vi "Abort Status Check.vi"(8 "error in (no error)":errorcluster, 11 "Guardian in":refnum<class "Guardian.lvclass">) -> (0 "error out":errorcluster, 3 "Guardian out":refnum<class "Guardian.lvclass">)   [LabVIEW 2026, in "TALOS.lvlib" / "Guardian.lvlib" / "Guardian.lvclass"]
doc: "This VI is called periodically to check the health status of ABORT and its unicity."
uses:
  Guardian.lvclass
  C:/LabVIEW Code/TALOS/talos/Ancestor/Ancestor/Ancestor.lvclass
  C:/LabVIEW Code/TALOS/builds/Actor Framework PPL/Actor Framework.lvlibp/1abvi3w/vi.lib/ActorFramework/Actor/Actor.lvclass
  Guardian.lvclass/Guardian.ctl
  Ancestor/Ancestor/Ancestor.lvclass/Ancestor.ctl
  Classes/Speedometer/Speedometer.lvclass/Speedometer.ctl
  Guardian Messages/Message to Other Guardian Msg/Message to Other Guardian Msg.lvclass/Message to Other Guardian Msg.ctl
  Guardian Messages/TCP-SV Message Interpreter Msg/TCP-SV Message Interpreter Msg.lvclass/TCP-SV Message Interpreter Msg.ctl
  4755b682-1248-473b-8cd2-dfaaffe09b65.vi
  cbc8a120-93e6-4d44-b253-7cefa591677c.vi
  3ae19a6a-4145-421c-a6fa-2879faec311c.vi
  Support VIs/Generate Error.vi
  <vilib>/Utility/High Resolution Relative Seconds.vi
  Broadcast to Guardians.vi
  FGV/Error Memory/Get Error Description.vi
  Support VIs/Get PC name.vi
  Support VIs/Get Class Name.vi
  Guardian Messages/Message to Other Guardian Msg/Send Message to Other Guardian.vi
  Support VIs/Search Array of Strings.vi
  Guardian Messages/TCP-SV Message Interpreter Msg/Send TCP-SV Message Interpreter.vi
  FGV/Error Memory/Error Memory Core.vi
  <vilib>/AdvancedString/Delimited String to 1D String Array.vi
  <vilib>/AdvancedString/Delimited String to 1D String Array (string).vi
  Support VIs/Circus Root Path.vi
  FGV/Error Memory/Error Crt Lvl checker.vi
  FGV/Error Memory/Error Memory Core.vi/40c8088d-b597-4017-91af-faa98e00292e.vi
  FGV/Error Memory/Error Memory Core.vi/d4a3ab98-063c-4e44-b43d-fbdcfe6c2be2.vi
  Support VIs/Global Memory.vi
  <vilib>/Utility/LVClass/Get LV Class Name.vi
  Support VIs/Is in Packed Library.vi
  Support VIs/TALOS Root path.vi
  Support VIs/Read CSV worksheet.vi
  Support VIs/Global Constants.vi
  <vilib>/Utility/error.llb/General Error Handler.vi
  <vilib>/Utility/config.llb/Open Config Data.vi
  <vilib>/Utility/config.llb/Get Section Names.vi
  <vilib>/Utility/config.llb/Get Key Names.vi
  <vilib>/Utility/config.llb/Read Key.vi
  <vilib>/Utility/config.llb/Read Key (String).vi
  <vilib>/Utility/config.llb/Close Config Data.vi
  Pat message.vi
  Support VIs/Circus Critical PCs List.vi
  builds/Actor Framework PPL/Actor Framework.lvlibp/1abvi3w/vi.lib/ActorFramework/Actor/Read Self Enqueuer.vi
  builds/Actor Framework PPL/Actor Framework.lvlibp/1abvi3w/vi.lib/ActorFramework/Message Enqueuer/Enqueue.vi
  Support VIs/Error Log.vi
  Support VIs/System Log.vi
  Ancestor/Ancestor/Ancestor.lvclass
  <vilib>/Comparison/Equal/Equal Functor/Equal Functor.lvclass
  Classes/Speedometer/Speedometer.lvclass
  <vilib>/Comparison/Less/Less Functor/Less Functor.lvclass
  Guardian Messages/Message to Other Guardian Msg/Message to Other Guardian Msg.lvclass
  Guardian Messages/TCP-SV Message Interpreter Msg/TCP-SV Message Interpreter Msg.lvclass
  Classes/Guardian List/Guardian List.lvclass
  TALOS.lvlib
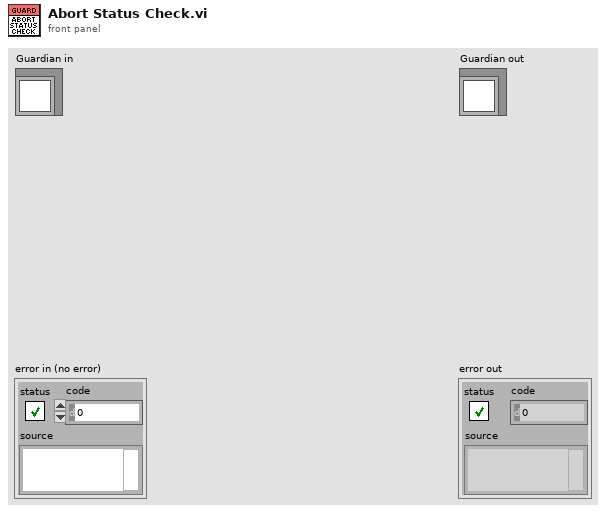
[diagram p1: front panel]
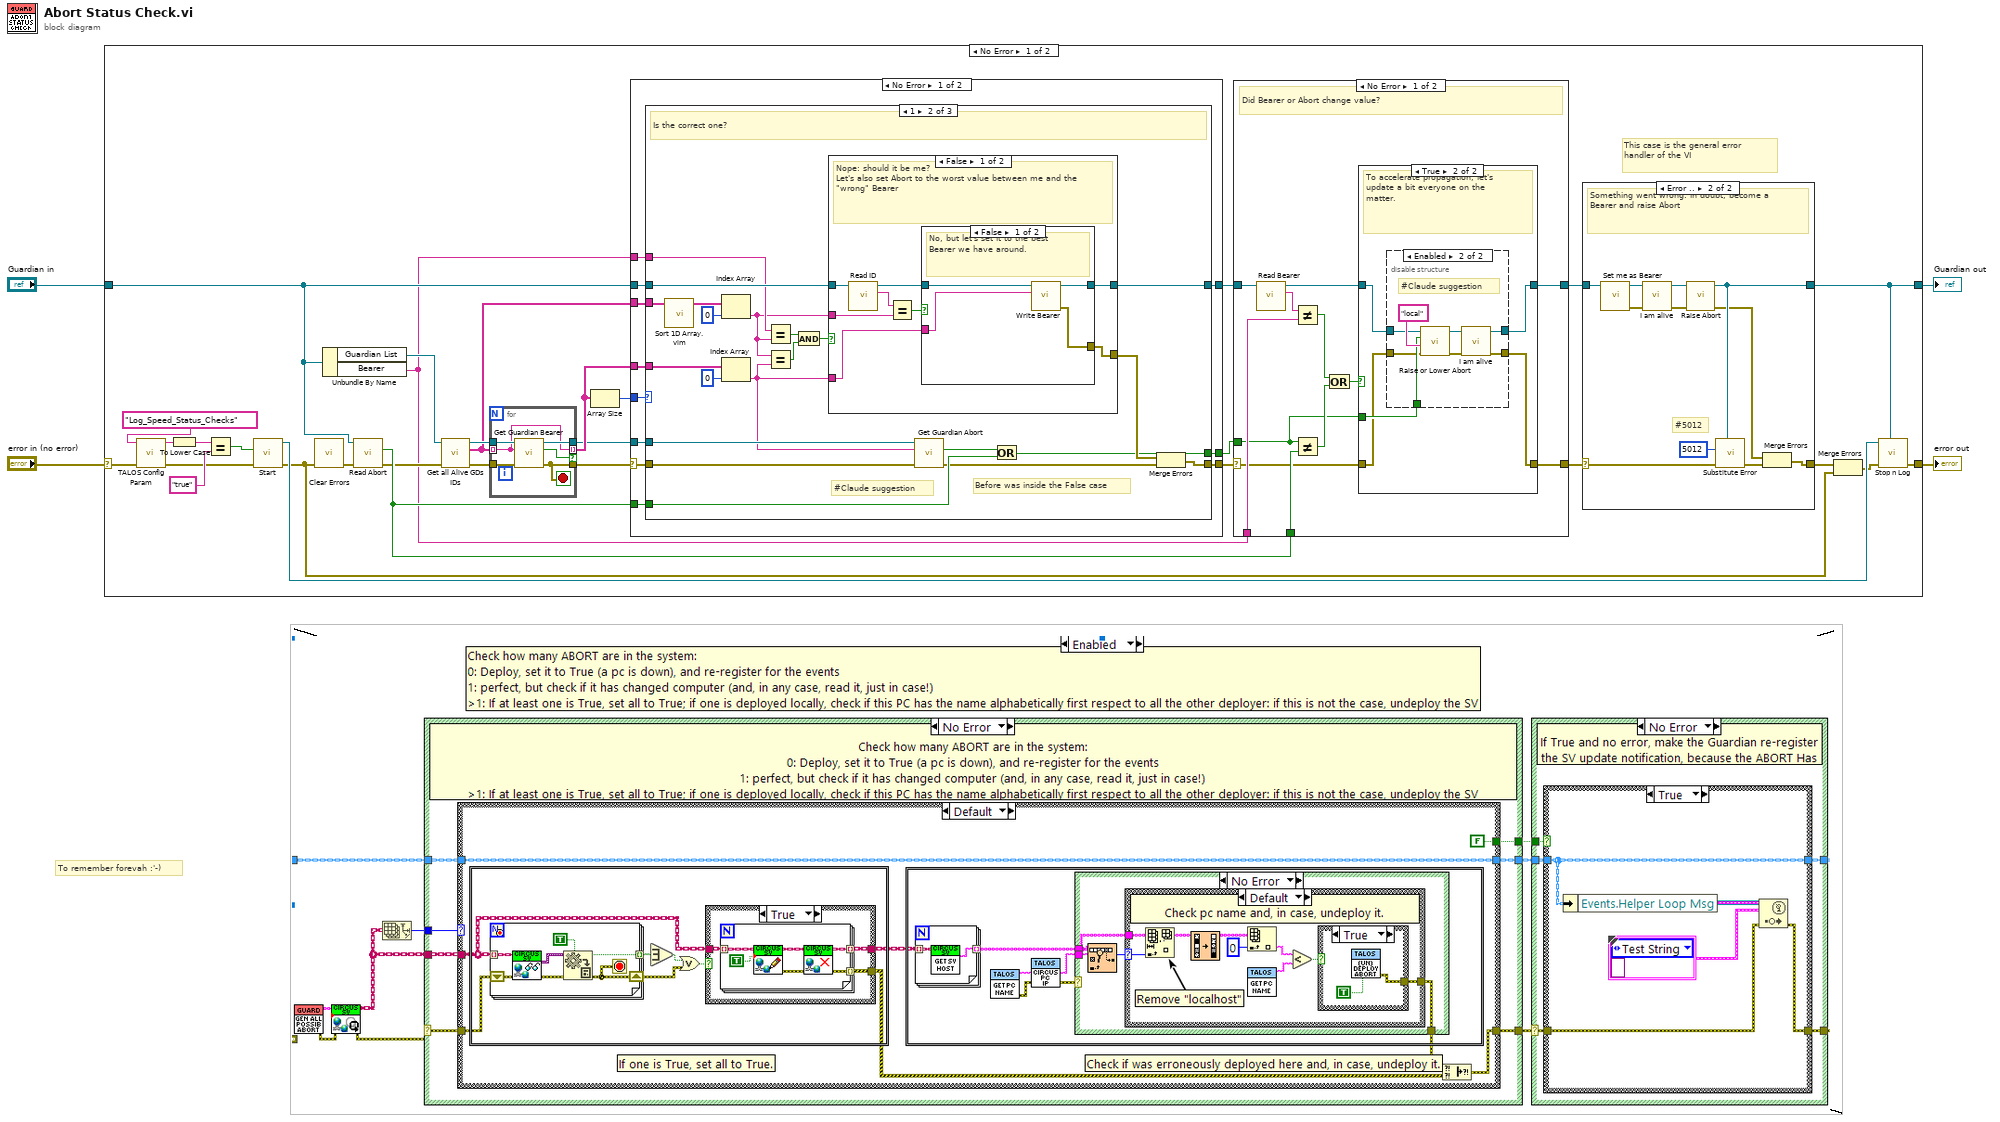
[diagram p0: block diagram]
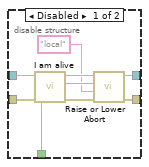
[diagram p3: hidden frame]
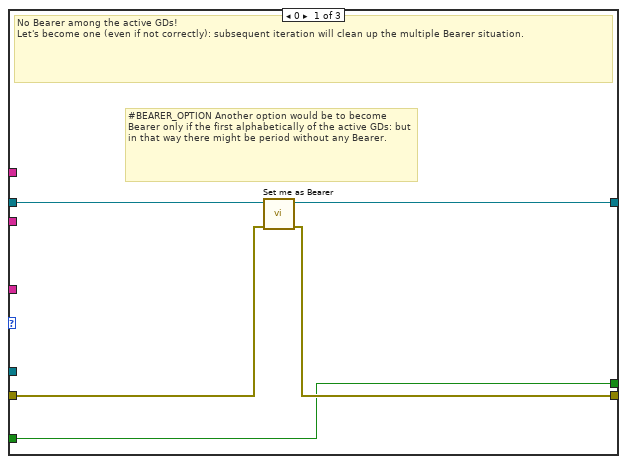
[diagram p5: hidden frame]
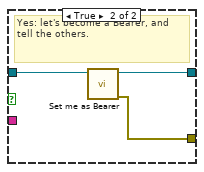
[diagram p6: hidden frame]
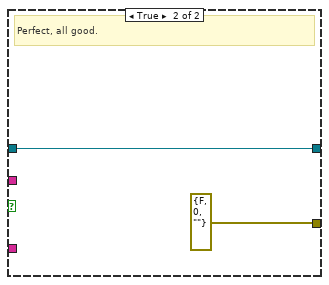
[diagram p7: hidden frame]
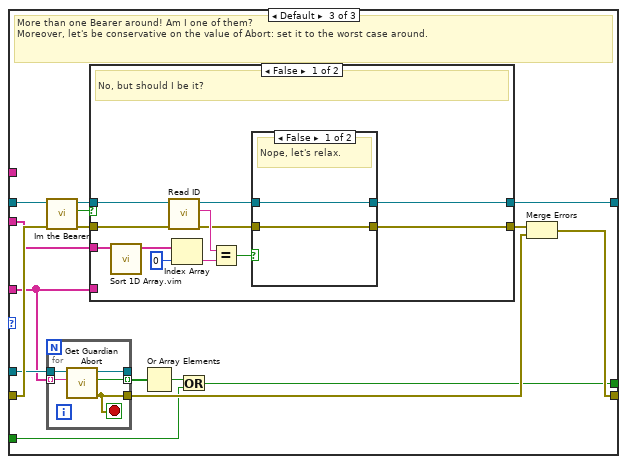
[diagram p8: hidden frame]
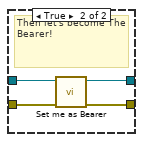
[diagram p9: hidden frame]
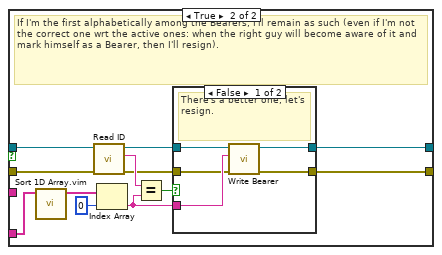
[diagram p10: hidden frame]
diagram:
  # "To remember forevah :'-)"
  n1 = case shown="No Error" "error in (no error)" {
    selector: "error in (no error)" -> [w25 w208]
    tunnel: [w34 w207] -> w1
    tunnel: [w33 w208] -> w3
    tunnel: "Guardian in" -> [w6 w207]
    frame No Error {
      # "This case is the general error handler of the VI"
      n2 = call "TALOS Config Param.vi"("error in (no error)"=w25, "Parameter Name"="Log_Speed_Status_Checks") -> ("error out"=w27:errorcluster, "Output"=w32:string)  [unwired: 8 in]
      n3 = To Lower Case(string=w32) -> (all lower case string=w31:string)
      n4 = Equal?(x=w31, y="true") -> (x = y?=w28:bool)
      n5 = call "Start.vi"("error in (no error)"=w27, "Active?"=w28) -> ("error out"=w23:errorcluster, "Speedometer out"=w35:refnum<class "Speedometer.lvclass">)  [unwired: 8 in]
      n6 = call <vilib>:"Clear Errors.vi"("error in (no error)"=w23) -> ("error out"=w9:errorcluster)  [unwired: 5 in, 1 out]
      n7 = Unbundle By Name(w6) -> ("Guardian List"=w20:refnum<class "Guardian List.lvclass">, "Bearer"=w5:string)
      n8 = call "Read Abort.vi"("error in (no error)"=w9, "Guardian in"=w6) -> ("error out"=w7:errorcluster, "Abort"=w8:bool)  [unwired: 7 in, 1 out]
      n9 = call-dynamic "Get all Alive GDs IDs.vi"("error in (no error)"=w7, "Guardian List in"=w20) -> ("error out"=w18:errorcluster, "Alive GDs IDs"=w15:string[], "Guardian List out"=w19:refnum<class "Guardian List.lvclass">)  [unwired: 7 in]
      n10 = for {
        tunnel: w19 -> [w192]
        tunnel: w15 -> [w189] mode=indexing
        tunnel: w18 -> [w193]
        tunnel: [w191] -> w13
        tunnel: [w190] -> w16
        tunnel: [w189] -> w14 mode=indexing if=w188
        stop <- w190 stop-if-true
        n11 = call-dynamic "Get Guardian Bearer.vi"("error in (no error)"=w193, "ID"=w189, "Guardian List in"=w192) -> ("error out"=w190:errorcluster, "Bearer"=w188:bool, "Guardian List out"=w191:refnum<class "Guardian List.lvclass">)  [unwired: 6 in]
      }
      n12 = Array Size(array=w14) -> (size(s)=w17:i32)
      n13 = case shown="No Error" w16 {
        selector: w16 -> [w82 w186]
        tunnel: w17 -> [w83 _]
        tunnel: w15 -> [w81 _]
        tunnel: w14 -> [w80 _]
        tunnel: w6 -> [w79 w187]
        tunnel: [w78 w187] -> w22
        tunnel: [w77 w186] -> w21
        tunnel: w13 -> [w76 _]
        tunnel: w8 -> [w75 w185]
        tunnel: [w74 w185] -> w10
        tunnel: w5 -> [w73 _]
        frame No Error {
          n14 = case shown="1" w83 {
            tunnel: w82 -> [w85 w107 w140]
            tunnel: w81 -> [_ w109 w134]
            tunnel: w80 -> [_ w108 w133]
            tunnel: w79 -> [w86 w106 w141]
            tunnel: [w88 w105 w130] -> w78
            tunnel: [w87 w97 w128] -> w77
            tunnel: w76 -> [_ w103 w136]
            tunnel: w75 -> [w84 w99 w131]
            tunnel: [w84 w98 w127] -> w74
            tunnel: w73 -> [_ w102 _]
            frame 0 {
              # "#BEARER_OPTION Another option would be to become Bearer only if the first alphabetically of the active GDs: but in that way there might be period without any Bearer."
              # "No Bearer among the active GDs!\nLet's become one (even if not correctly): subsequent iteration will clean up the multiple Bearer situation."
              n15 = call "Set me as Bearer.vi"("error in"=w85, "Guardian in"=w86) -> ("error out"=w87:errorcluster, "Guardian out"=w88:refnum<class "Guardian.lvclass">)  [unwired: 8 in]
            }
            frame 1 {
              # "Before was inside the False case"
              # "#Claude suggestion"
              # "Is the correct one?"
              n16 = call "Sort 1D Array.vim"("unsorted array"=w109) -> ("sorted array"=w95:string[])  [unwired: 10 in]
              n17 = Index Array(array=w95, index=0) -> (element=w90:string)
              n18 = Index Array(array=w108, index=0) -> (element=w101:string)
              n19 = Equal?(x=w102, y=w90) -> (x = y?=w92:bool)
              n20 = Equal?(x=w90, y=w101) -> (x = y?=w89:bool)
              n21 = And(x=w92, y=w89) -> (x .and. y?=w91:bool)
              n22 = case shown="False" w91 {
                tunnel: w106 -> [w117 w126]
                tunnel: w90 -> [w116 _]
                tunnel: [w112 w126] -> w105
                tunnel: [w111 errorcluster {"status"=FALSE, "code"=0, "source"=""} ("error out")] -> w104
                tunnel: w101 -> [w110 _]
                frame False {
                  # "Nope: should it be me?\nLet's also set Abort to the worst value between me and the \"wrong\" Bearer"
                  n23 = call "Read ID.vi"("Ancestor in"=w117) -> ("ID"=w113:string, "Ancestor out"=w114:refnum<class "Guardian.lvclass">)  [unwired: 8 in, 1 out]
                  n24 = Equal?(x=w113, y=w116) -> (x = y?=w115:bool)
                  n25 = case shown="False" w115 {
                    tunnel: w114 -> [w121 w124]
                    tunnel: [w120 w123] -> w112
                    tunnel: [w118 w122] -> w111
                    tunnel: w110 -> [w119 _]
                    frame False {
                      # "No, but let's set it to the best Bearer we have around."
                      n26 = call "Write Bearer.vi"("Bearer"=w119, "Guardian in"=w121) -> ("error out"=w118:errorcluster, "Guardian out"=w120:refnum<class "Guardian.lvclass">)  [unwired: 8 in]
                    }
                    frame True {
                      # "Yes: let's become a Bearer, and tell the others."
                      n27 = call "Set me as Bearer.vi"("Guardian in"=w124) -> ("error out"=w122:errorcluster, "Guardian out"=w123:refnum<class "Guardian.lvclass">)  [unwired: 9 in]
                    }
                  }
                }
                frame True {
                  # "Perfect, all good."
                }
              }
              n28 = call-dynamic "Get Guardian Abort.vi"("error in (no error)"=w107, "ID"=w101, "Guardian List in"=w103) -> ("error out"=w96:errorcluster, "Abort"=w100:bool)  [unwired: 6 in, 1 out]
              n29 = Or(x=w100, y=w99) -> (x .or. y?=w98:bool)
              n30 = Merge Errors(w104, w96) -> (w97:errorcluster)
            }
            frame Default {
              # "More than one Bearer around! Am I one of them?\nMoreover, let's be conservative on the value of Abort: set it to the worst case around."
              n31 = call "Im the Bearer.vi"("error in (no error)"=w140, "Guardian in"=w141) -> ("error out"=w139:errorcluster, "I'm the Bearer"=w138:bool, "Guardian out"=w137:refnum<class "Guardian.lvclass">)  [unwired: 7 in]
              n32 = for {
                tunnel: w136 -> [w147]
                tunnel: w133 -> [w146] mode=indexing
                tunnel: [w145] -> _
                tunnel: [w144] -> w135 mode=indexing
                tunnel: [w143] -> w142
                stop <- w143 stop-if-true
                n33 = call-dynamic "Get Guardian Abort.vi"("ID"=w146, "Guardian List in"=w147) -> ("error out"=w143:errorcluster, "Abort"=w144:bool, "Guardian List out"=w145:refnum<class "Guardian List.lvclass">)  [unwired: 7 in]
              }
              n34 = case shown="False" w138 {
                tunnel: w139 -> [w153 w173]
                tunnel: w137 -> [w155 w174]
                tunnel: w134 -> [w156 _]
                tunnel: w133 -> [_ w172]
                tunnel: [w149 w167] -> w130
                tunnel: [w148 w166] -> w129
                frame False {
                  # "No, but should I be it?"
                  n35 = call "Sort 1D Array.vim"("unsorted array"=w156) -> ("sorted array"=w159:string[])  [unwired: 10 in]
                  n36 = call "Read ID.vi"("error in (no error)"=w153, "Ancestor in"=w155) -> ("error out"=w151:errorcluster, "ID"=w157:string, "Ancestor out"=w150:refnum<class "Guardian.lvclass">)  [unwired: 7 in]
                  n37 = Index Array(array=w159, index=0) -> (element=w154:string)
                  n38 = Equal?(x=w157, y=w154) -> (x = y?=w152:bool)
                  n39 = case shown="False" w152 {
                    tunnel: w151 -> [w160 w164]
                    tunnel: w150 -> [w161 w165]
                    tunnel: [w161 w163] -> w149
                    tunnel: [w160 w162] -> w148
                    frame False {
                      # "Nope, let's relax."
                    }
                    frame True {
                      # "Then let's become The Bearer!"
                      n40 = call "Set me as Bearer.vi"("error in"=w164, "Guardian in"=w165) -> ("error out"=w162:errorcluster, "Guardian out"=w163:refnum<class "Guardian.lvclass">)  [unwired: 8 in]
                    }
                  }
                }
                frame True {
                  # "If I'm the first alphabetically among the Bearers, I'll remain as such (even if I'm not the correct one wrt the active ones: when the right guy will become aware of it and mark himself as a Bearer, then I'll resign)."
                  n41 = call "Sort 1D Array.vim"("unsorted array"=w172) -> ("sorted array"=w177:string[])  [unwired: 10 in]
                  n42 = call "Read ID.vi"("error in (no error)"=w173, "Ancestor in"=w174) -> ("error out"=w169:errorcluster, "ID"=w175:string, "Ancestor out"=w170:refnum<class "Guardian.lvclass">)  [unwired: 7 in]
                  n43 = Index Array(array=w177, index=0) -> (element=w168:string)
                  n44 = Equal?(x=w175, y=w168) -> (x = y?=w171:bool)
                  n45 = case shown="False" w171 {
                    tunnel: w170 -> [w182 w184]
                    tunnel: w169 -> [w180 w183]
                    tunnel: w168 -> [w181 _]
                    tunnel: [w179 w184] -> w167
                    tunnel: [w178 w183] -> w166
                    frame False {
                      # "There's a better one, let's resign."
                      n46 = call "Write Bearer.vi"("error in (no error)"=w180, "Bearer"=w181, "Guardian in"=w182) -> ("error out"=w178:errorcluster, "Guardian out"=w179:refnum<class "Guardian.lvclass">)  [unwired: 7 in]
                    }
                    frame True {
                      # "\"Most correct\" one possible."
                    }
                  }
                }
              }
              n47 = Or Array Elements(Boolean array=w135) -> (logical OR=w132:bool)
              n48 = Or(x=w132, y=w131) -> (x .or. y?=w127:bool)
              n49 = Merge Errors(w129, w142) -> (w128:errorcluster)
            }
          }
        }
        frame Error {
          # "It should never happen, but you know..."
        }
      }
      n50 = case shown="No Error" w21 {
        selector: w21 -> [w36 w71]
        tunnel: w22 -> [w47 w72]
        tunnel: w5 -> [w46 _]
        tunnel: w8 -> [w41 _]
        tunnel: [w39 w72] -> w12
        tunnel: [w38 w71] -> w11
        tunnel: w10 -> [w37 _]
        frame No Error {
          # "Did Bearer or Abort change value?"
          n51 = call "Read Bearer.vi"("Guardian in"=w47) -> ("Bearer"=w45:string, "Guardian out"=w40:refnum<class "Guardian.lvclass">)  [unwired: 8 in, 1 out]
          n52 = Not Equal?(x=w45, y=w46) -> (x != y?=w44:bool)
          n53 = Not Equal?(x=w37, y=w41) -> (x != y?=w43:bool)
          n54 = Or(x=w44, y=w43) -> (x .or. y?=w42:bool)
          n55 = case shown="True" w42 {
            tunnel: w36 -> [w48 w52]
            tunnel: w40 -> [w49 w54]
            tunnel: [w49 w50] -> w39
            tunnel: [w48 w51] -> w38
            tunnel: w37 -> [_ w53]
            frame False {
              # "Nothing changed, do nothing."
            }
            frame True {
              # "To accelerate propagation, let's update a bit everyone on the matter."
              n56 = disable-structure shown="Enabled" {
                disable-tunnel: w54 -> [w62 w69]
                disable-tunnel: w53 -> [w61 w68]
                disable-tunnel: w52 -> [w59 w67]
                disable-tunnel: [w57 w63] -> w51
                disable-tunnel: [w56 w65] -> w50
                frame Disabled {
                  n57 = call "I am alive.vi"("error in (no error)"=w59, "Guardian in"=w62) -> ("error out"=w58:errorcluster, "Guardian out"=w60:refnum<class "Guardian.lvclass">)  [unwired: 8 in]
                  n58 = call "Raise or Lower Abort.vi"("error in (no error)"=w58, "Sender"="local", "New Abort Value"=w61, "Guardian in"=w60) -> ("error out"=w57:errorcluster, "Guardian out"=w56:refnum<class "Guardian.lvclass">)  [unwired: 6 in]
                }
                frame Enabled {
                  # "#Claude suggestion"
                  n59 = call "Raise or Lower Abort.vi"("error in (no error)"=w67, "Sender"="local", "New Abort Value"=w68, "Guardian in"=w69) -> ("error out"=w64:errorcluster, "Guardian out"=w66:refnum<class "Guardian.lvclass">)  [unwired: 6 in]
                  n60 = call "I am alive.vi"("error in (no error)"=w64, "Guardian in"=w66) -> ("error out"=w63:errorcluster, "Guardian out"=w65:refnum<class "Guardian.lvclass">)  [unwired: 8 in]
                }
              }
            }
          }
        }
        frame Error {
          # "An error occurred, just go to the error handling of this VI."
        }
      }
      n61 = case shown="Error .." w11 {
        selector: w11 -> [w195 w201]
        tunnel: [w194 w200] -> w34
        tunnel: [w195 w197] -> w26
        tunnel: w12 -> [w194 w196]
        frame No Error {
          # "All good!"
        }
        frame Error {
          # "#5012"
          # "Something went wrong: in doubt, become a Bearer and raise Abort"
          n62 = call "Set me as Bearer.vi"("Guardian in"=w196) -> ("error out"=w203:errorcluster, "Guardian out"=w204:refnum<class "Guardian.lvclass">)  [unwired: 9 in]
          n63 = call "I am alive.vi"("error in (no error)"=w203, "Guardian in"=w204) -> ("error out"=w206:errorcluster, "Guardian out"=w205:refnum<class "Guardian.lvclass">)  [unwired: 8 in]
          n64 = call "Raise Abort.vi"("error in (no error)"=w206, "Guardian in"=w205) -> ("error out"=w199:errorcluster, "Guardian out"=w200:refnum<class "Guardian.lvclass">)  [unwired: 8 in]
          n65 = call "Substitute Error.vi"("LabVIEW Object"=w200, "error in (no error)"=w201, "Error Code"=5012) -> ("error out"=w198:errorcluster)  [unwired: 8 in]
          n66 = Merge Errors(w199, w198) -> (w197:errorcluster)
        }
      }
      n67 = Merge Errors(w26, w23) -> (w24:errorcluster)
      n68 = call "Stop n Log.vi"("Object in"=w34, "error in (no error)"=w24, "Speedometer in"=w35) -> ("error out"=w33:errorcluster)  [unwired: 8 in]
    }
    frame Error {
    }
  }
  "error out" <- w3
  "Guardian out" <- w1
